vi "例4.22 利用MATLAB脚本节点实现求和运算.vi"() -> ()   [LabVIEW 2017]
panel:
  out "sum":dbl
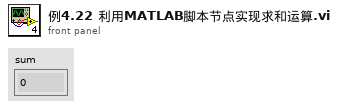
[diagram p1: front panel]
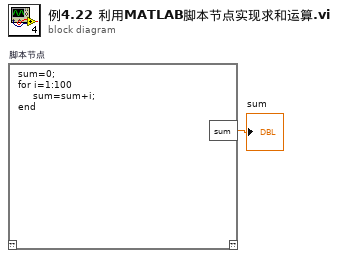
[diagram p0: block diagram]
diagram:
  n1 = script code="sum=0;\nfor i=1:100\n     sum=sum+i;\nend" "脚本节点"() -> ("sum"=→"sum":dbl)  [unwired: 1 in, 1 out]
